vi "TE_TemplateVIs.vi"() -> (3 "VI References":refnum<vi>[](array[refnum]))   [LabVIEW 2013, in "TemplateGenerator.lvlib"]
uses:
  TemplateGenerator.lvlib
  Current Value Table.lvlib
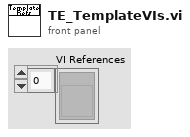
[diagram p1: front panel]
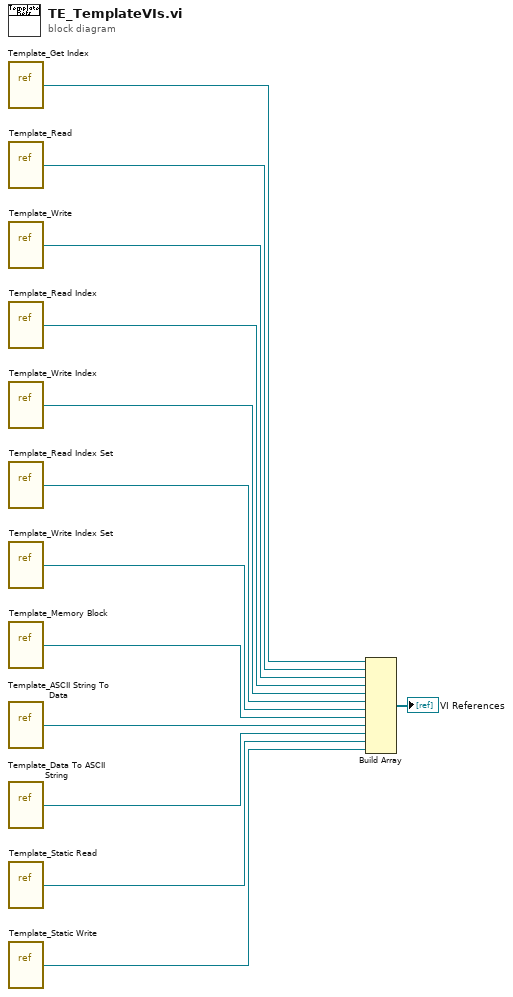
[diagram p0: block diagram]
diagram:
  n1 = vi-ref "Template_Get Index.vi"() -> (w12:refnum<vi>)
  n2 = vi-ref "Template_Read.vi"() -> (w11:refnum<vi>)
  n3 = vi-ref "Template_Write.vi"() -> (w10:refnum<vi>)
  n4 = vi-ref "Template_Read Index.vi"() -> (w9:refnum<vi>)
  n5 = vi-ref "Template_Write Index.vi"() -> (w8:refnum<vi>)
  n6 = vi-ref "Template_Read Index Set.vi"() -> (w7:refnum<vi>)
  n7 = vi-ref "Template_Write Index Set.vi"() -> (w5:refnum<vi>)
  n8 = vi-ref "Template_Memory Block.vi"() -> (w6:refnum<vi>)
  n9 = vi-ref "Template_ASCII String To Data.vi"() -> (w4:refnum<vi>)
  n10 = vi-ref "Template_Data To ASCII String.vi"() -> (w3:refnum<vi>)
  n11 = vi-ref "Template_Static Read.vi"() -> (w2:refnum<vi>)
  n12 = vi-ref "Template_Static Write.vi"() -> (w1:refnum<vi>)
  n13 = Build Array(w12, w11, w10, w9, w8, w7, w5, w6, w4, w3, w2, w1) -> (→"VI References":refnum<vi>[])
